vi "SP_OEE_2_test.vi"() -> ()   [LabVIEW 2017] (continued)
                            n1032 = call "Stack_holderwise_total_bd_count_&_duration.vi"("Refnum in"=w5667, "BREAKDOWN_STK_HOLD_ID"=5, "condition"=w5661, "Form Date"=w5664, "To Date"=w5665, "error in (no error)"=w5669) -> ("Refnum out"=w5666:T2, "Count out"=w5663:string[], "appended array"=w5662:dbl[], "error out"=w5668:errorcluster)  [unwired: 6 in]
                          }
                          frame Enabled {
                          }
                        }
                        n1033 = call "NUMERIC TO STRING.vi"("appended array"=w5641) -> ("Array"=w5640:string[])  [unwired: 4 in]
                        n1034 = call "Insert_empty_element_with_zero.vi"("searched date"=w5645, "fixed date"=w5643) -> ("O/P"=w5644:string[])  [unwired: 9 in]
                        n1035 = call "Insert_empty_element_with_zero.vi"("searched date"=w5640, "fixed date"=w5643) -> ("O/P"=w5642:string[])  [unwired: 9 in]
                      }
                      frame #6 {
                        n1036 = call "String to numeric.vi"("Array"=w5683) -> ("Array 2"=w5682:dbl[])  [unwired: 4 in]
                        n1037 = call "String to numeric.vi"("Array"=w5681) -> ("Array 2"=w5680:dbl[])  [unwired: 4 in]
                        n1038 = call "String to numeric.vi"("Array"=w5679) -> ("Array 2"=w5678:dbl[])  [unwired: 4 in]
                        n1039 = call "String to numeric.vi"("Array"=w5677) -> ("Array 2"=w5676:dbl[])  [unwired: 4 in]
                        n1040 = call "String to numeric.vi"("Array"=w5675) -> ("Array 2"=w5674:dbl[])  [unwired: 4 in]
                        n1041 = Decimal String To Number(string=w5688) -> (number=w5707:i32[])  [unwired: 2 in, 1 out]
                        n1042 = Decimal String To Number(string=w5689) -> (number=w5708:i32[])  [unwired: 2 in, 1 out]
                        n1043 = Decimal String To Number(string=w5690) -> (number=w5709:i32[])  [unwired: 2 in, 1 out]
                        n1044 = Decimal String To Number(string=w5691) -> (number=w5710:i32[])  [unwired: 2 in, 1 out]
                        n1045 = Decimal String To Number(string=w5692) -> (number=w5705:i32[])  [unwired: 2 in, 1 out]
                        n1046 = Compound Arithmetic op=ADD(w5682, w5680, w5678, w5676, w5674) -> (w5685:dbl[])
                        n1047 = Build Array(w5683) -> (w5704:string[][])
                        n1048 = Build Array(w5681) -> (w5703:string[][])
                        n1049 = Build Array(w5679) -> (w5702:string[][])
                        n1050 = Build Array(w5677) -> (w5701:string[][])
                        n1051 = Build Array(w5675) -> (w5700:string[][])
                        n1052 = Number To Fractional String(number=w5685, precision (6)=i16 2) -> (F-format string=w5684:string[])  [unwired: 2 in]
                        n1053 = Compound Arithmetic op=ADD(w5707, w5708, w5709, w5710, w5705) -> (w5711:i32[])
                        n1054 = Transpose 2D Array(2D array=w5704) -> (transposed array=w5698:string[][])
                        n1055 = Transpose 2D Array(2D array=w5703) -> (transposed array=w5697:string[][])
                        n1056 = Transpose 2D Array(2D array=w5702) -> (transposed array=w5696:string[][])
                        n1057 = Transpose 2D Array(2D array=w5701) -> (transposed array=w5695:string[][])
                        n1058 = Transpose 2D Array(2D array=w5700) -> (transposed array=w5694:string[][])
                        n1059 = Number To Decimal String(number=w5711) -> (decimal integer string=w5706:string[])  [unwired: 1 in]
                        n1060 = Build Array(w5684) -> (w5687:string[][])
                        n1061 = Transpose 2D Array(2D array=w5687) -> (transposed array=w5693:string[][])
                      }
                      frame #7 {
                        w5715 = string[] [""]
                        n1062 = Insert Into Array(array=w5724, index (col)=1 ("disabled index (col)"), new element #1=w5715, new element #2=w5715, new element #3=w5715, new element #4=w5715, new element #5=w5714, new element #6=w5716, new element #7=w5715, new element #8=w5715, new element #9=w5715, new element #10=w5715, new element #11=w5717, new element #12=w5718) -> (w5720:string[][])  [unwired: 1 in]
                        n1063 = call "flot graph for month n year.vi"("BD Date"=w5721, "error in (no error)"=w5723, "Count total"=w5717) -> ("error out"=w5722:errorcluster, "Run-Time Status"=w5719:cluster{"Array 2":timestamp[], dbl[]})  [unwired: 7 in]
                        n1064 = local write "Run-Time Status"(w5719) -> ()
                        n1065 = local write "Table"(w5720) -> ()
                      }
                    }
                  }
                  frame "3" {
                    n1066 = flat-sequence {
                      tunnel: w5735 -> [w5849]
                      tunnel: w5734 -> [w5847]
                      tunnel: [w5833] -> w5825
                      tunnel: [w5848] -> w5824
                      tunnel: w5733 -> [_]
                      tunnel: [w5852] -> w5823
                      tunnel: [w5832] -> w5822
                      tunnel: [w5831] -> w5821
                      tunnel: [w5830] -> w5820
                      tunnel: w5732 -> [w5832]
                      tunnel: w5731 -> [w5831]
                      tunnel: ["Where BREAKDOWN_DATE between '%s'and '%s' and BREAKDOWN_STK_HOLD_ID ='%d' and  SHIFT_ID = '%d' "] -> w5819
                      tunnel: [w5830] -> w5818
                      tunnel: w5730 -> [w5826]
                      tunnel: [w5826] -> w5729
                      tunnel: w5825 -> [w5913]
                      tunnel: w5824 -> [w5915]
                      tunnel: w5823 -> [w5911]
                      tunnel: w5822 -> [w5910]
                      tunnel: w5821 -> [w5909]
                      tunnel: [w5912] -> w5817
                      tunnel: [w5914] -> w5816
                      tunnel: [w5911] -> w5815
                      tunnel: [w5901] -> w5814
                      tunnel: [w5907] -> w5813
                      tunnel: [w5910] -> w5812
                      tunnel: [w5909] -> w5811
                      tunnel: w5820 -> [w5906]
                      tunnel: [w5906] -> w5810
                      tunnel: w5819 -> [w5903]
                      tunnel: [w5903] -> w5809
                      tunnel: [w5902] -> w5808
                      tunnel: w5818 -> [w5902]
                      tunnel: w5729 -> [w5900]
                      tunnel: [w5899] -> w5728
                      tunnel: w5817 -> [w5945]
                      tunnel: w5816 -> [w5943]
                      tunnel: w5815 -> [w5948]
                      tunnel: w5814 -> [w5947]
                      tunnel: w5813 -> [w5946]
                      tunnel: w5812 -> [w5941]
                      tunnel: w5811 -> [w5940]
                      tunnel: [w5948] -> w5807
                      tunnel: [w5947] -> w5806
                      tunnel: [w5946] -> w5805
                      tunnel: [w5944] -> w5804
                      tunnel: [w5938] -> w5803
                      tunnel: [w5937] -> w5802
                      tunnel: [w5942] -> w5801
                      tunnel: [w5941] -> w5800
                      tunnel: [w5940] -> w5799
                      tunnel: w5810 -> [w5936]
                      tunnel: [w5936] -> w5798
                      tunnel: w5809 -> [w5933]
                      tunnel: [w5933] -> w5797
                      tunnel: [w5932] -> w5796
                      tunnel: w5808 -> [w5932]
                      tunnel: w5728 -> [w5931]
                      tunnel: [w5930] -> w5727
                      tunnel: w5807 -> [w5983]
                      tunnel: w5806 -> [w5982]
                      tunnel: w5805 -> [w5981]
                      tunnel: w5804 -> [w5978]
                      tunnel: w5803 -> [w5980]
                      tunnel: w5802 -> [w5979]
                      tunnel: w5801 -> [w5976]
                      tunnel: w5800 -> [w5974]
                      tunnel: w5799 -> [w5973]
                      tunnel: [w5983] -> w5795
                      tunnel: [w5982] -> w5794
                      tunnel: [w5981] -> w5793
                      tunnel: [w5980] -> w5792
                      tunnel: [w5979] -> w5791
                      tunnel: [w5977] -> w5790
                      tunnel: [w5971] -> w5789
                      tunnel: [w5970] -> w5788
                      tunnel: [w5975] -> w5787
                      tunnel: [w5974] -> w5786
                      tunnel: [w5973] -> w5785
                      tunnel: w5798 -> [w5969]
                      tunnel: [w5969] -> w5784
                      tunnel: w5797 -> [w5966]
                      tunnel: [w5966] -> w5783
                      tunnel: [w5965] -> w5782
                      tunnel: w5796 -> [w5965]
                      tunnel: w5727 -> [w5963]
                      tunnel: w5795 -> [w6004]
                      tunnel: w5794 -> [w6003]
                      tunnel: w5793 -> [w6002]
                      tunnel: w5792 -> [w6001]
                      tunnel: w5791 -> [w6000]
                      tunnel: w5790 -> [w5997]
                      tunnel: w5789 -> [w5999]
                      tunnel: w5788 -> [w5998]
                      tunnel: w5787 -> [w5996]
                      tunnel: w5786 -> [w5993]
                      tunnel: w5785 -> [w5992]
                      tunnel: [w6004] -> w5781
                      tunnel: [w6003] -> w5780
                      tunnel: [w6002] -> w5779
                      tunnel: [w6001] -> w5778
                      tunnel: [w6000] -> w5777
                      tunnel: [w5999] -> w5776
                      tunnel: [w5998] -> w5775
                      tunnel: [w5995] -> w5774
                      tunnel: [w5994] -> w5773
                      tunnel: [w5990] -> w5772
                      tunnel: [w5989] -> w5771
                      tunnel: [w5993] -> w5770
                      tunnel: [w5992] -> w5769
                      tunnel: w5784 -> [w5988]
                      tunnel: [w5988] -> w5768
                      tunnel: w5783 -> [w5985]
                      tunnel: [w5985] -> w5767
                      tunnel: [w5984] -> w5766
                      tunnel: w5782 -> [w5984]
                      tunnel: w5781 -> [w6039]
                      tunnel: w5780 -> [w6038]
                      tunnel: w5779 -> [w6037]
                      tunnel: w5778 -> [w6036]
                      tunnel: w5777 -> [w6035]
                      tunnel: w5776 -> [w6034]
                      tunnel: w5775 -> [w6033]
                      tunnel: w5774 -> [w6028]
                      tunnel: w5773 -> [w6030]
                      tunnel: w5772 -> [w6032]
                      tunnel: w5771 -> [w6031]
                      tunnel: w5770 -> [w6025]
                      tunnel: w5769 -> [w6026]
                      tunnel: [w6039] -> w5765
                      tunnel: [w6038] -> w5764
                      tunnel: [w6037] -> w5763
                      tunnel: [w6036] -> w5762
                      tunnel: [w6035] -> w5761
                      tunnel: [w6034] -> w5760
                      tunnel: [w6033] -> w5759
                      tunnel: [w6032] -> w5758
                      tunnel: [w6031] -> w5757
                      tunnel: [w6029] -> w5756
                      tunnel: [w6027] -> w5755
                      tunnel: [w6023] -> w5754
                      tunnel: [w6021] -> w5753
                      tunnel: w5768 -> [w6022]
                      tunnel: w5767 -> [w6018]
                      tunnel: [w6017] -> w5752
                      tunnel: w5766 -> [w6017]
                      tunnel: w5765 -> [w6078]
                      tunnel: w5764 -> [w6071]
                      tunnel: w5763 -> [w6062]
                      tunnel: w5762 -> [w6070]
                      tunnel: w5761 -> [w6060]
                      tunnel: w5760 -> [w6069]
                      tunnel: w5759 -> [w6058]
                      tunnel: w5758 -> [w6068]
                      tunnel: w5757 -> [w6056]
                      tunnel: w5756 -> [w6092]
                      tunnel: w5755 -> [w6091]
                      tunnel: w5754 -> [w6067]
                      tunnel: w5753 -> [w6054]
                      tunnel: [w6092] -> w5751
                      tunnel: [w6091] -> w5750
                      tunnel: [w6085] -> w5749
                      tunnel: [w6078] -> w5748
                      tunnel: [w6077] -> w5747
                      tunnel: [w6076] -> w5746
                      tunnel: [w6075] -> w5745
                      tunnel: [w6074] -> w5744
                      tunnel: [w6073] -> w5743
                      tunnel: [w6072] -> w5742
                      tunnel: [w6071] -> w5741
                      tunnel: [w6070] -> w5740
                      tunnel: [w6069] -> w5739
                      tunnel: [w6068] -> w5738
                      tunnel: [w6067] -> w5737
                      tunnel: [w6052] -> w5736
                      tunnel: w5752 -> [w6052]
                      tunnel: [w6105] -> _
                      tunnel: [w6101] -> _
                      tunnel: w5751 -> [w6102]
                      tunnel: w5750 -> [w6105]
                      tunnel: w5749 -> [w6096]
                      tunnel: w5748 -> [w6103]
                      tunnel: w5747 -> [_]
                      tunnel: w5746 -> [_]
                      tunnel: w5745 -> [w6095]
                      tunnel: w5744 -> [_]
                      tunnel: w5743 -> [_]
                      tunnel: w5742 -> [w6097]
                      tunnel: w5741 -> [_]
                      tunnel: w5740 -> [_]
                      tunnel: w5739 -> [w6093]
                      tunnel: w5738 -> [_]
                      tunnel: w5737 -> [_]
                      tunnel: w5736 -> [w6100]
                      frame #0 {
                        w5840 = "%Y-%m-%d" ("time format string (%c)")
                        n1067 = Decimal String To Number(string=w5826) -> (number=w5827:i32)  [unwired: 2 in, 1 out]
                        n1068 = property on="Table" class="Tbl (strict)"("Visible"=TRUE) -> ()  [unwired: 2 in, 2 out]
                        n1069 = Format Date/Time String(time format string (%c)=w5840, seconds (now)=w5832) -> (date/time string=w5841:string)  [unwired: 1 in]
                        n1070 = Format Date/Time String(time format string (%c)=w5840, seconds (now)=w5831) -> (date/time string=w5839:string)  [unwired: 1 in]
                        n1071 = Format Into String(format string="Where BREAKDOWN_DATE between '%s' and '%s' and  SHIFT_ID = '%d'  ", w5841, w5839, w5827) -> (resulting string=w5838:string)  [unwired: 2 in, 1 out]
                        n1072 = call <vilib>:"DB Tools Select Data.vi"("condition"=w5838, "error in (no error)"=w5847, "columns"=string[] ["BREAKDOWN_DATE"], "table"="STATION_1_LOG_HISTORY", "connection reference"=w5849) -> ("error out"=w5834:errorcluster, "data"=w5837:variant[][], "connection reference out"=w5848:T2)  [unwired: 1 in]
                        n1073 = property on="Table 2" class="Tbl (strict)"("Visible"=FALSE) -> ()  [unwired: 2 in, 2 out]
                        n1074 = xnode "Database Variant To Data"("database variant"=w5837, "error in (no error)"=w5834, "type"=string[][] [] ("Elements Found")) -> ("data"=w5835:string[][], "error out"=w5833:errorcluster)
                        n1075 = Index Array(array=w5835, index (col)=0 ("disabled index (col)")) -> (element=w5843:string[])  [unwired: 1 in]
                        n1076 = call "Search_1d_array_element.vi"("Count in"=string[] [] ("Elements Found"), "BD Date"=w5843, "Elements Found in"=string[] [] ("Elements Found")) -> ("Elements Found out"=w5830:string[])  [unwired: 4 in, 2 out]
                        n1077 = Build Array(w5830) -> (w5853:string[][])
                        n1078 = Transpose 2D Array(2D array=w5853) -> (transposed array=w5852:string[][])
                      }
                      frame #1 {
                        n1079 = disable-structure shown="Enabled" {
                          disable-tunnel: w5915 -> [w5926 w5928]
                          disable-tunnel: [w5925 w5928] -> w5914
                          disable-tunnel: w5913 -> [w5924 w5929]
                          disable-tunnel: [w5923 w5929] -> w5912
                          disable-tunnel: w5910 -> [w5921 _]
                          disable-tunnel: w5909 -> [w5920 _]
                          disable-tunnel: [w5919 _] -> w5908
                          disable-tunnel: [w5918 _] -> w5905
                          disable-tunnel: w5903 -> [w5917 _]
                          disable-tunnel: w5900 -> [w5916 w5927]
                          disable-tunnel: [_ w5927] -> w5899
                          frame Disabled {
                            n1080 = call "Stack_holderwise_total_bd_count_&_duration_2.vi"("Refnum in"=w5926, "BREAKDOWN_STK_HOLD_ID"=1, "condition"=w5917, "Form Date"=w5921, "To Date"=w5920, "error in (no error)"=w5924, "Shift"=w5916) -> ("Refnum out"=w5925:T2, "Count out"=w5919:string[], "appended array"=w5918:dbl[], "error out"=w5923:errorcluster)  [unwired: 5 in]
                          }
                          frame Enabled {
                          }
                        }
                        n1081 = call "NUMERIC TO STRING.vi"("appended array"=w5905) -> ("Array"=w5904:string[])  [unwired: 4 in]
                        n1082 = call "Insert_empty_element_with_zero.vi"("searched date"=w5908, "fixed date"=w5906) -> ("O/P"=w5901:string[])  [unwired: 9 in]
                        n1083 = call "Insert_empty_element_with_zero.vi"("searched date"=w5904, "fixed date"=w5906) -> ("O/P"=w5907:string[])  [unwired: 9 in]
                      }
                      frame #2 {
                        n1084 = disable-structure shown="Enabled" {
                          disable-tunnel: w5945 -> [w5959 w5961]
                          disable-tunnel: [w5958 w5961] -> w5944
                          disable-tunnel: w5943 -> [w5957 w5962]
                          disable-tunnel: [w5956 w5962] -> w5942
                          disable-tunnel: w5941 -> [w5955 _]
                          disable-tunnel: w5940 -> [w5954 _]
                          disable-tunnel: [w5953 _] -> w5939
                          disable-tunnel: [w5952 _] -> w5935
                          disable-tunnel: w5933 -> [w5951 _]
                          disable-tunnel: w5931 -> [w5949 w5960]
                          disable-tunnel: [_ w5960] -> w5930
                          frame Disabled {
                            n1085 = call "Stack_holderwise_total_bd_count_&_duration_2.vi"("Refnum in"=w5957, "BREAKDOWN_STK_HOLD_ID"=2, "condition"=w5951, "Form Date"=w5955, "To Date"=w5954, "error in (no error)"=w5959, "Shift"=w5949) -> ("Refnum out"=w5956:T2, "Count out"=w5953:string[], "appended array"=w5952:dbl[], "error out"=w5958:errorcluster)  [unwired: 5 in]
                          }
                          frame Enabled {
                          }
                        }
                        n1086 = call "Insert_empty_element_with_zero.vi"("searched date"=w5939, "fixed date"=w5936) -> ("O/P"=w5938:string[])  [unwired: 9 in]
                        n1087 = call "NUMERIC TO STRING.vi"("appended array"=w5935) -> ("Array"=w5934:string[])  [unwired: 4 in]
                        n1088 = call "Insert_empty_element_with_zero.vi"("searched date"=w5934, "fixed date"=w5936) -> ("O/P"=w5937:string[])  [unwired: 9 in]
                      }
                      frame #3 {
                        n1089 = call "Stack_holderwise_total_bd_count_&_duration_2.vi"("Refnum in"=w5976, "BREAKDOWN_STK_HOLD_ID"=3, "condition"=w5966, "Form Date"=w5974, "To Date"=w5973, "error in (no error)"=w5978, "Shift"=w5963) -> ("Refnum out"=w5975:T2, "Count out"=w5972:string[], "appended array"=w5968:dbl[], "error out"=w5977:errorcluster)  [unwired: 5 in]
                        n1090 = call "Insert_empty_element_with_zero.vi"("searched date"=w5972, "fixed date"=w5969) -> ("O/P"=w5971:string[])  [unwired: 9 in]
                        n1091 = call "NUMERIC TO STRING.vi"("appended array"=w5968) -> ("Array"=w5967:string[])  [unwired: 4 in]
                        n1092 = call "Insert_empty_element_with_zero.vi"("searched date"=w5967, "fixed date"=w5969) -> ("O/P"=w5970:string[])  [unwired: 9 in]
                      }
                      frame #4 {
                        n1093 = disable-structure shown="Enabled" {
                          disable-tunnel: w5997 -> [w6013 w6016]
                          disable-tunnel: w5996 -> [w6012 w6015]
                          disable-tunnel: [w6011 w6015] -> w5995
                          disable-tunnel: [w6010 w6016] -> w5994
                          disable-tunnel: w5993 -> [w6009 _]
                          disable-tunnel: w5992 -> [w6008 _]
                          disable-tunnel: [w6007 _] -> w5991
                          disable-tunnel: [w6006 _] -> w5987
                          disable-tunnel: w5985 -> [w6005 _]
                          frame Disabled {
                            n1094 = call "Stack_holderwise_total_bd_count_&_duration.vi"("Refnum in"=w6012, "BREAKDOWN_STK_HOLD_ID"=4, "condition"=w6005, "Form Date"=w6009, "To Date"=w6008, "error in (no error)"=w6013) -> ("Refnum out"=w6011:T2, "Count out"=w6007:string[], "appended array"=w6006:dbl[], "error out"=w6010:errorcluster)  [unwired: 6 in]
                          }
                          frame Enabled {
                          }
                        }
                        n1095 = call "Insert_empty_element_with_zero.vi"("searched date"=w5991, "fixed date"=w5988) -> ("O/P"=w5990:string[])  [unwired: 9 in]
                        n1096 = call "NUMERIC TO STRING.vi"("appended array"=w5987) -> ("Array"=w5986:string[])  [unwired: 4 in]
                        n1097 = call "Insert_empty_element_with_zero.vi"("searched date"=w5986, "fixed date"=w5988) -> ("O/P"=w5989:string[])  [unwired: 9 in]
                      }
                      frame #5 {
                        n1098 = disable-structure shown="Enabled" {
                          disable-tunnel: w6030 -> [w6048 w6051]
                          disable-tunnel: [w6047 w6051] -> w6029
                          disable-tunnel: w6028 -> [w6046 w6050]
                          disable-tunnel: [w6045 w6050] -> w6027
                          disable-tunnel: w6026 -> [w6044 _]
                          disable-tunnel: w6025 -> [w6043 _]
                          disable-tunnel: [w6042 _] -> w6024
                          disable-tunnel: [w6041 _] -> w6020
                          disable-tunnel: w6018 -> [w6040 _]
                          frame Disabled {
                            n1099 = call "Stack_holderwise_total_bd_count_&_duration.vi"("Refnum in"=w6046, "BREAKDOWN_STK_HOLD_ID"=5, "condition"=w6040, "Form Date"=w6043, "To Date"=w6044, "error in (no error)"=w6048) -> ("Refnum out"=w6045:T2, "Count out"=w6042:string[], "appended array"=w6041:dbl[], "error out"=w6047:errorcluster)  [unwired: 6 in]
                          }
                          frame Enabled {
                          }
                        }
                        n1100 = call "NUMERIC TO STRING.vi"("appended array"=w6020) -> ("Array"=w6019:string[])  [unwired: 4 in]
                        n1101 = call "Insert_empty_element_with_zero.vi"("searched date"=w6024, "fixed date"=w6022) -> ("O/P"=w6023:string[])  [unwired: 9 in]
                        n1102 = call "Insert_empty_element_with_zero.vi"("searched date"=w6019, "fixed date"=w6022) -> ("O/P"=w6021:string[])  [unwired: 9 in]
                      }
                      frame #6 {
                        n1103 = call "String to numeric.vi"("Array"=w6062) -> ("Array 2"=w6061:dbl[])  [unwired: 4 in]
                        n1104 = call "String to numeric.vi"("Array"=w6060) -> ("Array 2"=w6059:dbl[])  [unwired: 4 in]
                        n1105 = call "String to numeric.vi"("Array"=w6058) -> ("Array 2"=w6057:dbl[])  [unwired: 4 in]
                        n1106 = call "String to numeric.vi"("Array"=w6056) -> ("Array 2"=w6055:dbl[])  [unwired: 4 in]
                        n1107 = call "String to numeric.vi"("Array"=w6054) -> ("Array 2"=w6053:dbl[])  [unwired: 4 in]
                        n1108 = Decimal String To Number(string=w6067) -> (number=w6086:i32[])  [unwired: 2 in, 1 out]
                        n1109 = Decimal String To Number(string=w6068) -> (number=w6087:i32[])  [unwired: 2 in, 1 out]
                        n1110 = Decimal String To Number(string=w6069) -> (number=w6088:i32[])  [unwired: 2 in, 1 out]
                        n1111 = Decimal String To Number(string=w6070) -> (number=w6089:i32[])  [unwired: 2 in, 1 out]
                        n1112 = Decimal String To Number(string=w6071) -> (number=w6084:i32[])  [unwired: 2 in, 1 out]
                        n1113 = Compound Arithmetic op=ADD(w6061, w6059, w6057, w6055, w6053) -> (w6064:dbl[])
                        n1114 = Build Array(w6062) -> (w6083:string[][])
                        n1115 = Build Array(w6060) -> (w6082:string[][])
                        n1116 = Build Array(w6058) -> (w6081:string[][])
                        n1117 = Build Array(w6056) -> (w6080:string[][])
                        n1118 = Build Array(w6054) -> (w6079:string[][])
                        n1119 = Number To Fractional String(number=w6064, precision (6)=i16 2) -> (F-format string=w6063:string[])  [unwired: 2 in]
                        n1120 = Compound Arithmetic op=ADD(w6086, w6087, w6088, w6089, w6084) -> (w6090:i32[])
                        n1121 = Transpose 2D Array(2D array=w6083) -> (transposed array=w6077:string[][])
                        n1122 = Transpose 2D Array(2D array=w6082) -> (transposed array=w6076:string[][])
                        n1123 = Transpose 2D Array(2D array=w6081) -> (transposed array=w6075:string[][])
                        n1124 = Transpose 2D Array(2D array=w6080) -> (transposed array=w6074:string[][])
                        n1125 = Transpose 2D Array(2D array=w6079) -> (transposed array=w6073:string[][])
                        n1126 = Number To Decimal String(number=w6090) -> (decimal integer string=w6085:string[])  [unwired: 1 in]
                        n1127 = Build Array(w6063) -> (w6066:string[][])
                        n1128 = Transpose 2D Array(2D array=w6066) -> (transposed array=w6072:string[][])
                      }
                      frame #7 {
                        w6094 = string[] [""]
                        n1129 = Insert Into Array(array=w6103, index (col)=1 ("disabled index (col)"), new element #1=w6094, new element #2=w6094, new element #3=w6094, new element #4=w6094, new element #5=w6093, new element #6=w6095, new element #7=w6094, new element #8=w6094, new element #9=w6094, new element #10=w6094, new element #11=w6096, new element #12=w6097) -> (w6099:string[][])  [unwired: 1 in]
                        n1130 = call "flot graph for month n year.vi"("BD Date"=w6100, "error in (no error)"=w6102, "Count total"=w6096) -> ("error out"=w6101:errorcluster, "Run-Time Status"=w6098:cluster{"Array 2":timestamp[], dbl[]})  [unwired: 7 in]
                        n1131 = local write "Run-Time Status"(w6098) -> ()
                        n1132 = local write "Table"(w6099) -> ()
                      }
                    }
                  }
                  frame "all" {
                  }
                }
              }
              frame "Quality" {
                n1133 = local read "Shift"() -> (w6106:string)
                n1134 = case shown="\"3\"" w6106 {
                  selector: w6106 -> [_ w6480 w6864 w7248 _]
                  tunnel: w6111 -> [w6116 w6485 w6869 w7253 _]
                  tunnel: w6110 -> [w6115 w6484 w6868 w7252 _]
                  tunnel: w6109 -> [w6114 w6483 w6867 w7251 _]
                  tunnel: w6108 -> [w6113 w6482 w6866 w7250 _]
                  tunnel: w6107 -> [w6112 w6481 w6865 w7249 _]
                  frame "ALL", Default {
                    n1135 = flat-sequence {
                      tunnel: w6116 -> [w6228]
                      tunnel: w6115 -> [w6226]
                      tunnel: [w6212] -> w6206
                      tunnel: [w6227] -> w6205
                      tunnel: w6114 -> [_]
                      tunnel: [w6231] -> w6204
                      tunnel: [w6211] -> w6203
                      tunnel: [w6210] -> w6202
                      tunnel: [w6208] -> w6201
                      tunnel: w6113 -> [w6211]
                      tunnel: w6112 -> [w6210]
                      tunnel: ["Where BREAKDOWN_DATE between '%s'and '%s' and BREAKDOWN_STK_HOLD_ID ='%d'  "] -> w6200
                      tunnel: [w6208] -> w6199
                      tunnel: w6206 -> [w6290]
                      tunnel: w6205 -> [w6292]
                      tunnel: w6204 -> [w6288]
                      tunnel: w6203 -> [w6287]
                      tunnel: w6202 -> [w6286]
                      tunnel: [w6289] -> w6198
                      tunnel: [w6291] -> w6197
                      tunnel: [w6288] -> w6196
                      tunnel: [w6278] -> w6195
                      tunnel: [w6284] -> w6194
                      tunnel: [w6287] -> w6193
                      tunnel: [w6286] -> w6192
                      tunnel: w6201 -> [w6283]
                      tunnel: [w6283] -> w6191
                      tunnel: w6200 -> [w6280]
                      tunnel: [w6280] -> w6190
                      tunnel: [w6279] -> w6189
                      tunnel: w6199 -> [w6279]
                      tunnel: w6198 -> [w6318]
                      tunnel: w6197 -> [w6316]
                      tunnel: w6196 -> [w6321]
                      tunnel: w6195 -> [w6320]
                      tunnel: w6194 -> [w6319]
                      tunnel: w6193 -> [w6314]
                      tunnel: w6192 -> [w6313]
                      tunnel: [w6321] -> w6188
                      tunnel: [w6320] -> w6187
                      tunnel: [w6319] -> w6186
                      tunnel: [w6317] -> w6185
                      tunnel: [w6311] -> w6184
                      tunnel: [w6310] -> w6183
                      tunnel: [w6315] -> w6182
                      tunnel: [w6314] -> w6181
                      tunnel: [w6313] -> w6180
                      tunnel: w6191 -> [w6309]
                      tunnel: [w6309] -> w6179
                      tunnel: w6190 -> [w6306]
                      tunnel: [w6306] -> w6178
                      tunnel: [w6305] -> w6177
                      tunnel: w6189 -> [w6305]
                      tunnel: w6188 -> [w6352]
                      tunnel: w6187 -> [w6351]
                      tunnel: w6186 -> [w6350]
                      tunnel: w6185 -> [w6347]
                      tunnel: w6184 -> [w6349]
                      tunnel: w6183 -> [w6348]
                      tunnel: w6182 -> [w6345]
                      tunnel: w6181 -> [w6343]
                      tunnel: w6180 -> [w6342]
                      tunnel: [w6352] -> w6176
                      tunnel: [w6351] -> w6175
                      tunnel: [w6350] -> w6174
                      tunnel: [w6349] -> w6173
                      tunnel: [w6348] -> w6172
                      tunnel: [w6346] -> w6171
                      tunnel: [w6340] -> w6170
                      tunnel: [w6339] -> w6169
                      tunnel: [w6344] -> w6168
                      tunnel: [w6343] -> w6167
                      tunnel: [w6342] -> w6166
                      tunnel: w6179 -> [w6338]
                      tunnel: [w6338] -> w6165
                      tunnel: w6178 -> [w6335]
                      tunnel: [w6335] -> w6164
                      tunnel: [w6334] -> w6163
                      tunnel: w6177 -> [w6334]
                      tunnel: w6176 -> [w6386]
                      tunnel: w6175 -> [w6385]
                      tunnel: w6174 -> [w6384]
                      tunnel: w6173 -> [w6383]
                      tunnel: w6172 -> [w6382]
                      tunnel: w6171 -> [w6379]
                      tunnel: w6170 -> [w6381]
                      tunnel: w6169 -> [w6380]
                      tunnel: w6168 -> [w6378]
                      tunnel: w6167 -> [w6375]
                      tunnel: w6166 -> [w6374]
                      tunnel: [w6386] -> w6162
                      tunnel: [w6385] -> w6161
                      tunnel: [w6384] -> w6160
                      tunnel: [w6383] -> w6159
                      tunnel: [w6382] -> w6158
                      tunnel: [w6381] -> w6157
                      tunnel: [w6380] -> w6156
                      tunnel: [w6377] -> w6155
                      tunnel: [w6376] -> w6154
                      tunnel: [w6372] -> w6153
                      tunnel: [w6371] -> w6152
                      tunnel: [w6375] -> w6151
                      tunnel: [w6374] -> w6150
                      tunnel: w6165 -> [w6370]
                      tunnel: [w6370] -> w6149
                      tunnel: w6164 -> [w6367]
                      tunnel: [w6367] -> w6148
                      tunnel: [w6366] -> w6147
                      tunnel: w6163 -> [w6366]
                      tunnel: w6162 -> [w6409]
                      tunnel: w6161 -> [w6408]
                      tunnel: w6160 -> [w6407]
                      tunnel: w6159 -> [w6406]
                      tunnel: w6158 -> [w6405]
                      tunnel: w6157 -> [w6404]
                      tunnel: w6156 -> [w6403]
                      tunnel: w6155 -> [w6398]
                      tunnel: w6154 -> [w6400]
                      tunnel: w6153 -> [w6402]
                      tunnel: w6152 -> [w6401]
                      tunnel: w6151 -> [w6395]
                      tunnel: w6150 -> [w6396]
                      tunnel: [w6409] -> w6146
                      tunnel: [w6408] -> w6145
                      tunnel: [w6407] -> w6144
                      tunnel: [w6406] -> w6143
                      tunnel: [w6405] -> w6142
                      tunnel: [w6404] -> w6141
                      tunnel: [w6403] -> w6140
                      tunnel: [w6402] -> w6139
                      tunnel: [w6401] -> w6138
                      tunnel: [w6399] -> w6137
                      tunnel: [w6397] -> w6136
                      tunnel: [w6393] -> w6135
                      tunnel: [w6391] -> w6134
                      tunnel: w6149 -> [w6392]
                      tunnel: w6148 -> [w6388]
                      tunnel: [w6387] -> w6133
                      tunnel: w6147 -> [w6387]
                      tunnel: w6146 -> [w6448]
                      tunnel: w6145 -> [w6441]
                      tunnel: w6144 -> [w6432]
                      tunnel: w6143 -> [w6440]
                      tunnel: w6142 -> [w6430]
                      tunnel: w6141 -> [w6439]
                      tunnel: w6140 -> [w6428]
                      tunnel: w6139 -> [w6438]
                      tunnel: w6138 -> [w6426]
                      tunnel: w6137 -> [w6462]
                      tunnel: w6136 -> [w6461]
                      tunnel: w6135 -> [w6437]
                      tunnel: w6134 -> [w6424]
                      tunnel: [w6462] -> w6132
                      tunnel: [w6461] -> w6131
                      tunnel: [w6455] -> w6130
                      tunnel: [w6448] -> w6129
                      tunnel: [w6447] -> w6128
                      tunnel: [w6446] -> w6127
                      tunnel: [w6445] -> w6126
                      tunnel: [w6444] -> w6125
                      tunnel: [w6443] -> w6124
                      tunnel: [w6442] -> w6123
                      tunnel: [w6441] -> w6122
                      tunnel: [w6440] -> w6121
                      tunnel: [w6439] -> w6120
                      tunnel: [w6438] -> w6119
                      tunnel: [w6437] -> w6118
                      tunnel: [w6422] -> w6117
                      tunnel: w6133 -> [w6422]
                      tunnel: [w6475] -> _
                      tunnel: [w6471] -> _
                      tunnel: w6132 -> [w6472]
                      tunnel: w6131 -> [w6475]
                      tunnel: w6130 -> [w6466]
                      tunnel: w6129 -> [w6473]
                      tunnel: w6128 -> [_]
                      tunnel: w6127 -> [_]
                      tunnel: w6126 -> [_]
                      tunnel: w6125 -> [w6463]
                      tunnel: w6124 -> [_]
                      tunnel: w6123 -> [w6467]
                      tunnel: w6122 -> [_]
                      tunnel: w6121 -> [_]
                      tunnel: w6120 -> [_]
                      tunnel: w6119 -> [w6464]
                      tunnel: w6118 -> [_]
                      tunnel: w6117 -> [w6470]
                      frame #0 {
                        w6219 = "%Y-%m-%d" ("time format string (%c)")
                        n1136 = property on="Table" class="Tbl (strict)"("Visible"=TRUE) -> ()  [unwired: 2 in, 2 out]
                        n1137 = Format Date/Time String(time format string (%c)=w6219, seconds (now)=w6211) -> (date/time string=w6220:string)  [unwired: 1 in]
                        n1138 = Format Date/Time String(time format string (%c)=w6219, seconds (now)=w6210) -> (date/time string=w6218:string)  [unwired: 1 in]
                        n1139 = Format Into String(format string="Where BREAKDOWN_DATE between '%s' and '%s' ", w6220, w6218) -> (resulting string=w6217:string)  [unwired: 2 in, 1 out]
                        n1140 = call <vilib>:"DB Tools Select Data.vi"("condition"=w6217, "error in (no error)"=w6226, "columns"=string[] ["BREAKDOWN_DATE"], "table"="STATION_1_LOG_HISTORY", "connection reference"=w6228) -> ("error out"=w6213:errorcluster, "data"=w6216:variant[][], "connection reference out"=w6227:T2)  [unwired: 1 in]
                        n1141 = property on="Table 2" class="Tbl (strict)"("Visible"=FALSE) -> ()  [unwired: 2 in, 2 out]
                        n1142 = xnode "Database Variant To Data"("database variant"=w6216, "error in (no error)"=w6213, "type"=string[][] [] ("Elements Found")) -> ("data"=w6214:string[][], "error out"=w6212:errorcluster)
                        n1143 = Index Array(array=w6214, index (col)=0 ("disabled index (col)")) -> (element=w6222:string[])  [unwired: 1 in]
                        n1144 = call "Search_1d_array_element.vi"("Count in"=string[] [] ("Elements Found"), "BD Date"=w6222, "Elements Found in"=string[] [] ("Elements Found")) -> ("Elements Found out"=w6208:string[])  [unwired: 4 in, 2 out]
                        n1145 = Build Array(w6208) -> (w6232:string[][])
                        n1146 = Transpose 2D Array(2D array=w6232) -> (transposed array=w6231:string[][])
                      }
                      frame #1 {
                        n1147 = disable-structure shown="Enabled" {
                          disable-tunnel: w6292 -> [w6302 w6303]
                          disable-tunnel: [w6301 w6303] -> w6291
                          disable-tunnel: w6290 -> [w6300 w6304]
                          disable-tunnel: [w6299 w6304] -> w6289
                          disable-tunnel: w6287 -> [w6297 _]
                          disable-tunnel: w6286 -> [w6296 _]
                          disable-tunnel: [w6295 _] -> w6285
                          disable-tunnel: [w6294 _] -> w6282
                          disable-tunnel: w6280 -> [w6293 _]
                          frame Disabled {
                            n1148 = call "Stack_holderwise_total_bd_count_&_duration.vi"("Refnum in"=w6302, "BREAKDOWN_STK_HOLD_ID"=1, "condition"=w6293, "Form Date"=w6297, "To Date"=w6296, "error in (no error)"=w6300) -> ("Refnum out"=w6301:T2, "Count out"=w6295:string[], "appended array"=w6294:dbl[], "error out"=w6299:errorcluster)  [unwired: 6 in]
                          }
                          frame Enabled {
                          }
                        }
                        n1149 = call "NUMERIC TO STRING.vi"("appended array"=w6282) -> ("Array"=w6281:string[])  [unwired: 4 in]
                        n1150 = call "Insert_empty_element_with_zero.vi"("searched date"=w6285, "fixed date"=w6283) -> ("O/P"=w6278:string[])  [unwired: 9 in]
                        n1151 = call "Insert_empty_element_with_zero.vi"("searched date"=w6281, "fixed date"=w6283) -> ("O/P"=w6284:string[])  [unwired: 9 in]
                      }
                      frame #2 {
                        n1152 = disable-structure shown="Enabled" {
                          disable-tunnel: w6318 -> [w6331 w6333]
                          disable-tunnel: [w6330 w6333] -> w6317
                          disable-tunnel: w6316 -> [w6329 w6332]
                          disable-tunnel: [w6328 w6332] -> w6315
                          disable-tunnel: w6314 -> [w6327 _]
                          disable-tunnel: w6313 -> [w6326 _]
                          disable-tunnel: [w6325 _] -> w6312
                          disable-tunnel: [w6324 _] -> w6308
                          disable-tunnel: w6306 -> [w6323 _]
                          frame Disabled {
                            n1153 = call "Stack_holderwise_total_bd_count_&_duration.vi"("Refnum in"=w6329, "BREAKDOWN_STK_HOLD_ID"=2, "condition"=w6323, "Form Date"=w6327, "To Date"=w6326, "error in (no error)"=w6331) -> ("Refnum out"=w6328:T2, "Count out"=w6325:string[], "appended array"=w6324:dbl[], "error out"=w6330:errorcluster)  [unwired: 6 in]
                          }
                          frame Enabled {
                          }
                        }
                        n1154 = call "Insert_empty_element_with_zero.vi"("searched date"=w6312, "fixed date"=w6309) -> ("O/P"=w6311:string[])  [unwired: 9 in]
                        n1155 = call "NUMERIC TO STRING.vi"("appended array"=w6308) -> ("Array"=w6307:string[])  [unwired: 4 in]
                        n1156 = call "Insert_empty_element_with_zero.vi"("searched date"=w6307, "fixed date"=w6309) -> ("O/P"=w6310:string[])  [unwired: 9 in]
                      }
                      frame #3 {
                        n1157 = disable-structure shown="Enabled" {
                          disable-tunnel: w6347 -> [w6362 w6364]
                          disable-tunnel: [w6361 w6364] -> w6346
                          disable-tunnel: w6345 -> [w6360 w6363]
                          disable-tunnel: [w6359 w6363] -> w6344
                          disable-tunnel: w6343 -> [w6358 _]
                          disable-tunnel: w6342 -> [w6357 _]
                          disable-tunnel: [w6356 _] -> w6341
                          disable-tunnel: [w6355 _] -> w6337
                          disable-tunnel: w6335 -> [w6354 _]
                          frame Disabled {
                            n1158 = call "Stack_holderwise_total_bd_count_&_duration.vi"("Refnum in"=w6360, "BREAKDOWN_STK_HOLD_ID"=3, "condition"=w6354, "Form Date"=w6358, "To Date"=w6357, "error in (no error)"=w6362) -> ("Refnum out"=w6359:T2, "Count out"=w6356:string[], "appended array"=w6355:dbl[], "error out"=w6361:errorcluster)  [unwired: 6 in]
                          }
                          frame Enabled {
                          }
                        }
                        n1159 = call "Insert_empty_element_with_zero.vi"("searched date"=w6341, "fixed date"=w6338) -> ("O/P"=w6340:string[])  [unwired: 9 in]
                        n1160 = call "NUMERIC TO STRING.vi"("appended array"=w6337) -> ("Array"=w6336:string[])  [unwired: 4 in]
                        n1161 = call "Insert_empty_element_with_zero.vi"("searched date"=w6336, "fixed date"=w6338) -> ("O/P"=w6339:string[])  [unwired: 9 in]
                      }
                      frame #4 {
                        n1162 = call "Stack_holderwise_total_bd_count_&_duration.vi"("Refnum in"=w6378, "BREAKDOWN_STK_HOLD_ID"=4, "condition"=w6367, "Form Date"=w6375, "To Date"=w6374, "error in (no error)"=w6379) -> ("Refnum out"=w6377:T2, "Count out"=w6373:string[], "appended array"=w6369:dbl[], "error out"=w6376:errorcluster)  [unwired: 6 in]
                        n1163 = call "Insert_empty_element_with_zero.vi"("searched date"=w6373, "fixed date"=w6370) -> ("O/P"=w6372:string[])  [unwired: 9 in]
                        n1164 = call "NUMERIC TO STRING.vi"("appended array"=w6369) -> ("Array"=w6368:string[])  [unwired: 4 in]
                        n1165 = call "Insert_empty_element_with_zero.vi"("searched date"=w6368, "fixed date"=w6370) -> ("O/P"=w6371:string[])  [unwired: 9 in]
                      }
                      frame #5 {
                        n1166 = disable-structure shown="Enabled" {
                          disable-tunnel: w6400 -> [w6418 w6421]
                          disable-tunnel: [w6417 w6421] -> w6399
                          disable-tunnel: w6398 -> [w6416 w6420]
                          disable-tunnel: [w6415 w6420] -> w6397
                          disable-tunnel: w6396 -> [w6414 _]
                          disable-tunnel: w6395 -> [w6413 _]
                          disable-tunnel: [w6412 _] -> w6394
                          disable-tunnel: [w6411 _] -> w6390
                          disable-tunnel: w6388 -> [w6410 _]
                          frame Disabled {
                            n1167 = call "Stack_holderwise_total_bd_count_&_duration.vi"("Refnum in"=w6416, "BREAKDOWN_STK_HOLD_ID"=5, "condition"=w6410, "Form Date"=w6413, "To Date"=w6414, "error in (no error)"=w6418) -> ("Refnum out"=w6415:T2, "Count out"=w6412:string[], "appended array"=w6411:dbl[], "error out"=w6417:errorcluster)  [unwired: 6 in]
                          }
                          frame Enabled {
                          }
                        }
                        n1168 = call "NUMERIC TO STRING.vi"("appended array"=w6390) -> ("Array"=w6389:string[])  [unwired: 4 in]
                        n1169 = call "Insert_empty_element_with_zero.vi"("searched date"=w6394, "fixed date"=w6392) -> ("O/P"=w6393:string[])  [unwired: 9 in]
                        n1170 = call "Insert_empty_element_with_zero.vi"("searched date"=w6389, "fixed date"=w6392) -> ("O/P"=w6391:string[])  [unwired: 9 in]
                      }
                      frame #6 {
                        n1171 = call "String to numeric.vi"("Array"=w6432) -> ("Array 2"=w6431:dbl[])  [unwired: 4 in]
                        n1172 = call "String to numeric.vi"("Array"=w6430) -> ("Array 2"=w6429:dbl[])  [unwired: 4 in]
                        n1173 = call "String to numeric.vi"("Array"=w6428) -> ("Array 2"=w6427:dbl[])  [unwired: 4 in]
                        n1174 = call "String to numeric.vi"("Array"=w6426) -> ("Array 2"=w6425:dbl[])  [unwired: 4 in]
                        n1175 = call "String to numeric.vi"("Array"=w6424) -> ("Array 2"=w6423:dbl[])  [unwired: 4 in]
                        n1176 = Decimal String To Number(string=w6437) -> (number=w6456:i32[])  [unwired: 2 in, 1 out]
                        n1177 = Decimal String To Number(string=w6438) -> (number=w6457:i32[])  [unwired: 2 in, 1 out]
                        n1178 = Decimal String To Number(string=w6439) -> (number=w6458:i32[])  [unwired: 2 in, 1 out]
                        n1179 = Decimal String To Number(string=w6440) -> (number=w6459:i32[])  [unwired: 2 in, 1 out]
                        n1180 = Decimal String To Number(string=w6441) -> (number=w6454:i32[])  [unwired: 2 in, 1 out]
                        n1181 = Compound Arithmetic op=ADD(w6431, w6429, w6427, w6425, w6423) -> (w6434:dbl[])
                        n1182 = Build Array(w6432) -> (w6453:string[][])
                        n1183 = Build Array(w6430) -> (w6452:string[][])
                        n1184 = Build Array(w6428) -> (w6451:string[][])
                        n1185 = Build Array(w6426) -> (w6450:string[][])
                        n1186 = Build Array(w6424) -> (w6449:string[][])
                        n1187 = Number To Fractional String(number=w6434, precision (6)=i16 2) -> (F-format string=w6433:string[])  [unwired: 2 in]
                        n1188 = Compound Arithmetic op=ADD(w6456, w6457, w6458, w6459, w6454) -> (w6460:i32[])
                        n1189 = Transpose 2D Array(2D array=w6453) -> (transposed array=w6447:string[][])
                        n1190 = Transpose 2D Array(2D array=w6452) -> (transposed array=w6446:string[][])
                        n1191 = Transpose 2D Array(2D array=w6451) -> (transposed array=w6445:string[][])
                        n1192 = Transpose 2D Array(2D array=w6450) -> (transposed array=w6444:string[][])
                        n1193 = Transpose 2D Array(2D array=w6449) -> (transposed array=w6443:string[][])
                        n1194 = Number To Decimal String(number=w6460) -> (decimal integer string=w6455:string[])  [unwired: 1 in]
                        n1195 = Build Array(w6433) -> (w6436:string[][])
                        n1196 = Transpose 2D Array(2D array=w6436) -> (transposed array=w6442:string[][])
                      }
                      frame #7 {
                        w6465 = string[] [""]
                        n1197 = Insert Into Array(array=w6473, index (col)=1 ("disabled index (col)"), new element #1=w6465, new element #2=w6465, new element #3=w6465, new element #4=w6465, new element #5=w6465, new element #6=w6465, new element #7=w6464, new element #8=w6463, new element #9=w6465, new element #10=w6465, new element #11=w6466, new element #12=w6467) -> (w6469:string[][])  [unwired: 1 in]
                        n1198 = call "flot graph for month n year.vi"("BD Date"=w6470, "error in (no error)"=w6472, "Count total"=w6466) -> ("error out"=w6471:errorcluster, "Run-Time Status"=w6468:cluster{"Array 2":timestamp[], dbl[]})  [unwired: 7 in]
                        n1199 = local write "Run-Time Status"(w6468) -> ()
                        n1200 = local write "Table"(w6469) -> ()
                      }
                    }
                  }
                  frame "1" {
                    n1201 = flat-sequence {
                      tunnel: w6485 -> [w6599]
                      tunnel: w6484 -> [w6597]
                      tunnel: [w6583] -> w6575
                      tunnel: [w6598] -> w6574
                      tunnel: w6483 -> [_]
                      tunnel: [w6602] -> w6573
                      tunnel: [w6582] -> w6572
                      tunnel: [w6581] -> w6571
                      tunnel: [w6580] -> w6570
                      tunnel: w6482 -> [w6582]
                      tunnel: w6481 -> [w6581]
                      tunnel: ["Where BREAKDOWN_DATE between '%s'and '%s' and BREAKDOWN_STK_HOLD_ID ='%d' and  SHIFT_ID = '%d' "] -> w6569
                      tunnel: [w6580] -> w6568
                      tunnel: w6480 -> [w6576]
                      tunnel: [w6576] -> w6479
                      tunnel: w6575 -> [w6663]
                      tunnel: w6574 -> [w6665]
                      tunnel: w6573 -> [w6661]
                      tunnel: w6572 -> [w6660]
                      tunnel: w6571 -> [w6659]
                      tunnel: [w6662] -> w6567
                      tunnel: [w6664] -> w6566
                      tunnel: [w6661] -> w6565
                      tunnel: [w6651] -> w6564
                      tunnel: [w6657] -> w6563
                      tunnel: [w6660] -> w6562
                      tunnel: [w6659] -> w6561
                      tunnel: w6570 -> [w6656]
                      tunnel: [w6656] -> w6560
                      tunnel: w6569 -> [w6653]
                      tunnel: [w6653] -> w6559
                      tunnel: [w6652] -> w6558
                      tunnel: w6568 -> [w6652]
                      tunnel: w6479 -> [w6650]
                      tunnel: [w6649] -> w6478
                      tunnel: w6567 -> [w6695]
                      tunnel: w6566 -> [w6693]
                      tunnel: w6565 -> [w6698]
                      tunnel: w6564 -> [w6697]
                      tunnel: w6563 -> [w6696]
                      tunnel: w6562 -> [w6691]
                      tunnel: w6561 -> [w6690]
                      tunnel: [w6698] -> w6557
                      tunnel: [w6697] -> w6556
                      tunnel: [w6696] -> w6555
                      tunnel: [w6694] -> w6554
                      tunnel: [w6688] -> w6553
                      tunnel: [w6687] -> w6552
                      tunnel: [w6692] -> w6551
                      tunnel: [w6691] -> w6550
                      tunnel: [w6690] -> w6549
                      tunnel: w6560 -> [w6686]
                      tunnel: [w6686] -> w6548
                      tunnel: w6559 -> [w6683]
                      tunnel: [w6683] -> w6547
                      tunnel: [w6682] -> w6546
                      tunnel: w6558 -> [w6682]
                      tunnel: w6478 -> [w6681]
                      tunnel: [w6680] -> w6477
                      tunnel: w6557 -> [w6733]
                      tunnel: w6556 -> [w6732]
                      tunnel: w6555 -> [w6731]
                      tunnel: w6554 -> [w6728]
                      tunnel: w6553 -> [w6730]
                      tunnel: w6552 -> [w6729]
                      tunnel: w6551 -> [w6726]
                      tunnel: w6550 -> [w6724]
                      tunnel: w6549 -> [w6723]
                      tunnel: [w6733] -> w6545
                      tunnel: [w6732] -> w6544
                      tunnel: [w6731] -> w6543
                      tunnel: [w6730] -> w6542
                      tunnel: [w6729] -> w6541
                      tunnel: [w6727] -> w6540
                      tunnel: [w6721] -> w6539
                      tunnel: [w6720] -> w6538
                      tunnel: [w6725] -> w6537
                      tunnel: [w6724] -> w6536
                      tunnel: [w6723] -> w6535
                      tunnel: w6548 -> [w6719]
                      tunnel: [w6719] -> w6534
                      tunnel: w6547 -> [w6716]
                      tunnel: [w6716] -> w6533
                      tunnel: [w6715] -> w6532
                      tunnel: w6546 -> [w6715]
                      tunnel: w6477 -> [w6714]
                      tunnel: [w6713] -> w6476
                      tunnel: w6545 -> [w6770]
                      tunnel: w6544 -> [w6769]
                      tunnel: w6543 -> [w6768]
                      tunnel: w6542 -> [w6767]
                      tunnel: w6541 -> [w6766]
                      tunnel: w6540 -> [w6763]
                      tunnel: w6539 -> [w6765]
                      tunnel: w6538 -> [w6764]
                      tunnel: w6537 -> [w6762]
                      tunnel: w6536 -> [w6759]
                      tunnel: w6535 -> [w6758]
                      tunnel: [w6770] -> w6531
                      tunnel: [w6769] -> w6530
                      tunnel: [w6768] -> w6529
                      tunnel: [w6767] -> w6528
                      tunnel: [w6766] -> w6527
                      tunnel: [w6765] -> w6526
                      tunnel: [w6764] -> w6525
                      tunnel: [w6761] -> w6524
                      tunnel: [w6760] -> w6523
                      tunnel: [w6756] -> w6522
                      tunnel: [w6755] -> w6521
                      tunnel: [w6759] -> w6520
                      tunnel: [w6758] -> w6519
                      tunnel: w6534 -> [w6754]
                      tunnel: [w6754] -> w6518
                      tunnel: w6533 -> [w6751]
                      tunnel: [w6751] -> w6517
                      tunnel: [w6750] -> w6516
                      tunnel: w6532 -> [w6750]
                      tunnel: w6476 -> [w6748]
                      tunnel: w6531 -> [w6793]
                      tunnel: w6530 -> [w6792]
                      tunnel: w6529 -> [w6791]
                      tunnel: w6528 -> [w6790]
                      tunnel: w6527 -> [w6789]
                      tunnel: w6526 -> [w6788]
                      tunnel: w6525 -> [w6787]
                      tunnel: w6524 -> [w6782]
                      tunnel: w6523 -> [w6784]
                      tunnel: w6522 -> [w6786]
                      tunnel: w6521 -> [w6785]
                      tunnel: w6520 -> [w6779]
                      tunnel: w6519 -> [w6780]
                      tunnel: [w6793] -> w6515
                      tunnel: [w6792] -> w6514
                      tunnel: [w6791] -> w6513
                      tunnel: [w6790] -> w6512
                      tunnel: [w6789] -> w6511
                      tunnel: [w6788] -> w6510
                      tunnel: [w6787] -> w6509
                      tunnel: [w6786] -> w6508
                      tunnel: [w6785] -> w6507
                      tunnel: [w6783] -> w6506
                      tunnel: [w6781] -> w6505
                      tunnel: [w6777] -> w6504
                      tunnel: [w6775] -> w6503
                      tunnel: w6518 -> [w6776]
                      tunnel: w6517 -> [w6772]
                      tunnel: [w6771] -> w6502
                      tunnel: w6516 -> [w6771]
                      tunnel: w6515 -> [w6832]
                      tunnel: w6514 -> [w6825]
                      tunnel: w6513 -> [w6816]
                      tunnel: w6512 -> [w6824]
                      tunnel: w6511 -> [w6814]
                      tunnel: w6510 -> [w6823]
                      tunnel: w6509 -> [w6812]
                      tunnel: w6508 -> [w6822]
                      tunnel: w6507 -> [w6810]
                      tunnel: w6506 -> [w6846]
                      tunnel: w6505 -> [w6845]
                      tunnel: w6504 -> [w6821]
                      tunnel: w6503 -> [w6808]
                      tunnel: [w6846] -> w6501
                      tunnel: [w6845] -> w6500
                      tunnel: [w6839] -> w6499
                      tunnel: [w6832] -> w6498
                      tunnel: [w6831] -> w6497
                      tunnel: [w6830] -> w6496
                      tunnel: [w6829] -> w6495
                      tunnel: [w6828] -> w6494
                      tunnel: [w6827] -> w6493
                      tunnel: [w6826] -> w6492
                      tunnel: [w6825] -> w6491
                      tunnel: [w6824] -> w6490
                      tunnel: [w6823] -> w6489
                      tunnel: [w6822] -> w6488
                      tunnel: [w6821] -> w6487
                      tunnel: [w6806] -> w6486
                      tunnel: w6502 -> [w6806]
                      tunnel: [w6859] -> _
                      tunnel: [w6855] -> _
                      tunnel: w6501 -> [w6856]
                      tunnel: w6500 -> [w6859]
                      tunnel: w6499 -> [w6850]
                      tunnel: w6498 -> [w6857]
                      tunnel: w6497 -> [_]
                      tunnel: w6496 -> [_]
                      tunnel: w6495 -> [_]
                      tunnel: w6494 -> [w6847]
                      tunnel: w6493 -> [_]
                      tunnel: w6492 -> [w6851]
                      tunnel: w6491 -> [_]
                      tunnel: w6490 -> [_]
                      tunnel: w6489 -> [_]
                      tunnel: w6488 -> [w6848]
                      tunnel: w6487 -> [_]
                      tunnel: w6486 -> [w6854]
                      frame #0 {
                        w6590 = "%Y-%m-%d" ("time format string (%c)")
                        n1202 = Decimal String To Number(string=w6576) -> (number=w6577:i32)  [unwired: 2 in, 1 out]
                        n1203 = property on="Table" class="Tbl (strict)"("Visible"=TRUE) -> ()  [unwired: 2 in, 2 out]
                        n1204 = Format Date/Time String(time format string (%c)=w6590, seconds (now)=w6582) -> (date/time string=w6591:string)  [unwired: 1 in]
                        n1205 = Format Date/Time String(time format string (%c)=w6590, seconds (now)=w6581) -> (date/time string=w6589:string)  [unwired: 1 in]
                        n1206 = Format Into String(format string="Where BREAKDOWN_DATE between '%s' and '%s' and  SHIFT_ID = '%d'  ", w6591, w6589, w6577) -> (resulting string=w6588:string)  [unwired: 2 in, 1 out]
                        n1207 = call <vilib>:"DB Tools Select Data.vi"("condition"=w6588, "error in (no error)"=w6597, "columns"=string[] ["BREAKDOWN_DATE"], "table"="STATION_1_LOG_HISTORY", "connection reference"=w6599) -> ("error out"=w6584:errorcluster, "data"=w6587:variant[][], "connection reference out"=w6598:T2)  [unwired: 1 in]
                        n1208 = property on="Table 2" class="Tbl (strict)"("Visible"=FALSE) -> ()  [unwired: 2 in, 2 out]
                        n1209 = xnode "Database Variant To Data"("database variant"=w6587, "error in (no error)"=w6584, "type"=string[][] [] ("Elements Found")) -> ("data"=w6585:string[][], "error out"=w6583:errorcluster)
                        n1210 = Index Array(array=w6585, index (col)=0 ("disabled index (col)")) -> (element=w6593:string[])  [unwired: 1 in]
                        n1211 = call "Search_1d_array_element.vi"("Count in"=string[] [] ("Elements Found"), "BD Date"=w6593, "Elements Found in"=string[] [] ("Elements Found")) -> ("Elements Found out"=w6580:string[])  [unwired: 4 in, 2 out]
                        n1212 = Build Array(w6580) -> (w6603:string[][])
                        n1213 = Transpose 2D Array(2D array=w6603) -> (transposed array=w6602:string[][])
                      }
                      frame #1 {
                        n1214 = disable-structure shown="Enabled" {
                          disable-tunnel: w6665 -> [w6676 w6678]
                          disable-tunnel: [w6675 w6678] -> w6664
                          disable-tunnel: w6663 -> [w6674 w6679]
                          disable-tunnel: [w6673 w6679] -> w6662
                          disable-tunnel: w6660 -> [w6671 _]
                          disable-tunnel: w6659 -> [w6670 _]
                          disable-tunnel: [w6669 _] -> w6658
                          disable-tunnel: [w6668 _] -> w6655
                          disable-tunnel: w6653 -> [w6667 _]
                          disable-tunnel: w6650 -> [w6666 w6677]
                          disable-tunnel: [_ w6677] -> w6649
                          frame Disabled {
                            n1215 = call "Stack_holderwise_total_bd_count_&_duration_2.vi"("Refnum in"=w6676, "BREAKDOWN_STK_HOLD_ID"=1, "condition"=w6667, "Form Date"=w6671, "To Date"=w6670, "error in (no error)"=w6674, "Shift"=w6666) -> ("Refnum out"=w6675:T2, "Count out"=w6669:string[], "appended array"=w6668:dbl[], "error out"=w6673:errorcluster)  [unwired: 5 in]
                          }
                          frame Enabled {
                          }
                        }
                        n1216 = call "NUMERIC TO STRING.vi"("appended array"=w6655) -> ("Array"=w6654:string[])  [unwired: 4 in]
                        n1217 = call "Insert_empty_element_with_zero.vi"("searched date"=w6658, "fixed date"=w6656) -> ("O/P"=w6651:string[])  [unwired: 9 in]
                        n1218 = call "Insert_empty_element_with_zero.vi"("searched date"=w6654, "fixed date"=w6656) -> ("O/P"=w6657:string[])  [unwired: 9 in]
                      }
                      frame #2 {
                        n1219 = disable-structure shown="Enabled" {
                          disable-tunnel: w6695 -> [w6709 w6711]
                          disable-tunnel: [w6708 w6711] -> w6694
                          disable-tunnel: w6693 -> [w6707 w6712]
                          disable-tunnel: [w6706 w6712] -> w6692
                          disable-tunnel: w6691 -> [w6705 _]
                          disable-tunnel: w6690 -> [w6704 _]
                          disable-tunnel: [w6703 _] -> w6689
                          disable-tunnel: [w6702 _] -> w6685
                          disable-tunnel: w6683 -> [w6701 _]
                          disable-tunnel: w6681 -> [w6699 w6710]
                          disable-tunnel: [_ w6710] -> w6680
                          frame Disabled {
                            n1220 = call "Stack_holderwise_total_bd_count_&_duration_2.vi"("Refnum in"=w6707, "BREAKDOWN_STK_HOLD_ID"=2, "condition"=w6701, "Form Date"=w6705, "To Date"=w6704, "error in (no error)"=w6709, "Shift"=w6699) -> ("Refnum out"=w6706:T2, "Count out"=w6703:string[], "appended array"=w6702:dbl[], "error out"=w6708:errorcluster)  [unwired: 5 in]
                          }
                          frame Enabled {
                          }
                        }
                        n1221 = call "Insert_empty_element_with_zero.vi"("searched date"=w6689, "fixed date"=w6686) -> ("O/P"=w6688:string[])  [unwired: 9 in]
                        n1222 = call "NUMERIC TO STRING.vi"("appended array"=w6685) -> ("Array"=w6684:string[])  [unwired: 4 in]
                        n1223 = call "Insert_empty_element_with_zero.vi"("searched date"=w6684, "fixed date"=w6686) -> ("O/P"=w6687:string[])  [unwired: 9 in]
                      }
                      frame #3 {
                        n1224 = disable-structure shown="Enabled" {
                          disable-tunnel: w6728 -> [w6744 w6746]
                          disable-tunnel: [w6743 w6746] -> w6727
                          disable-tunnel: w6726 -> [w6742 w6747]
                          disable-tunnel: [w6741 w6747] -> w6725
                          disable-tunnel: w6724 -> [w6740 _]
                          disable-tunnel: w6723 -> [w6739 _]
                          disable-tunnel: [w6738 _] -> w6722
                          disable-tunnel: [w6737 _] -> w6718
                          disable-tunnel: w6716 -> [w6736 _]
                          disable-tunnel: w6714 -> [w6734 w6745]
                          disable-tunnel: [_ w6745] -> w6713
                          frame Disabled {
                            n1225 = call "Stack_holderwise_total_bd_count_&_duration_2.vi"("Refnum in"=w6742, "BREAKDOWN_STK_HOLD_ID"=3, "condition"=w6736, "Form Date"=w6740, "To Date"=w6739, "error in (no error)"=w6744, "Shift"=w6734) -> ("Refnum out"=w6741:T2, "Count out"=w6738:string[], "appended array"=w6737:dbl[], "error out"=w6743:errorcluster)  [unwired: 5 in]
                          }
                          frame Enabled {
                          }
                        }
                        n1226 = call "Insert_empty_element_with_zero.vi"("searched date"=w6722, "fixed date"=w6719) -> ("O/P"=w6721:string[])  [unwired: 9 in]
                        n1227 = call "NUMERIC TO STRING.vi"("appended array"=w6718) -> ("Array"=w6717:string[])  [unwired: 4 in]
                        n1228 = call "Insert_empty_element_with_zero.vi"("searched date"=w6717, "fixed date"=w6719) -> ("O/P"=w6720:string[])  [unwired: 9 in]
                      }
                      frame #4 {
                        n1229 = call "Stack_holderwise_total_bd_count_&_duration_2.vi"("Refnum in"=w6762, "BREAKDOWN_STK_HOLD_ID"=4, "condition"=w6751, "Form Date"=w6759, "To Date"=w6758, "error in (no error)"=w6763, "Shift"=w6748) -> ("Refnum out"=w6761:T2, "Count out"=w6757:string[], "appended array"=w6753:dbl[], "error out"=w6760:errorcluster)  [unwired: 5 in]
                        n1230 = call "Insert_empty_element_with_zero.vi"("searched date"=w6757, "fixed date"=w6754) -> ("O/P"=w6756:string[])  [unwired: 9 in]
                        n1231 = call "NUMERIC TO STRING.vi"("appended array"=w6753) -> ("Array"=w6752:string[])  [unwired: 4 in]
                        n1232 = call "Insert_empty_element_with_zero.vi"("searched date"=w6752, "fixed date"=w6754) -> ("O/P"=w6755:string[])  [unwired: 9 in]
                      }
                      frame #5 {
                        n1233 = disable-structure shown="Enabled" {
                          disable-tunnel: w6784 -> [w6802 w6805]
                          disable-tunnel: [w6801 w6805] -> w6783
                          disable-tunnel: w6782 -> [w6800 w6804]
                          disable-tunnel: [w6799 w6804] -> w6781
                          disable-tunnel: w6780 -> [w6798 _]
                          disable-tunnel: w6779 -> [w6797 _]
                          disable-tunnel: [w6796 _] -> w6778
                          disable-tunnel: [w6795 _] -> w6774
                          disable-tunnel: w6772 -> [w6794 _]
                          frame Disabled {
                            n1234 = call "Stack_holderwise_total_bd_count_&_duration.vi"("Refnum in"=w6800, "BREAKDOWN_STK_HOLD_ID"=5, "condition"=w6794, "Form Date"=w6797, "To Date"=w6798, "error in (no error)"=w6802) -> ("Refnum out"=w6799:T2, "Count out"=w6796:string[], "appended array"=w6795:dbl[], "error out"=w6801:errorcluster)  [unwired: 6 in]
                          }
                          frame Enabled {
                          }
                        }
                        n1235 = call "NUMERIC TO STRING.vi"("appended array"=w6774) -> ("Array"=w6773:string[])  [unwired: 4 in]
                        n1236 = call "Insert_empty_element_with_zero.vi"("searched date"=w6778, "fixed date"=w6776) -> ("O/P"=w6777:string[])  [unwired: 9 in]
                        n1237 = call "Insert_empty_element_with_zero.vi"("searched date"=w6773, "fixed date"=w6776) -> ("O/P"=w6775:string[])  [unwired: 9 in]
                      }
                      frame #6 {
                        n1238 = call "String to numeric.vi"("Array"=w6816) -> ("Array 2"=w6815:dbl[])  [unwired: 4 in]
                        n1239 = call "String to numeric.vi"("Array"=w6814) -> ("Array 2"=w6813:dbl[])  [unwired: 4 in]
                        n1240 = call "String to numeric.vi"("Array"=w6812) -> ("Array 2"=w6811:dbl[])  [unwired: 4 in]
                        n1241 = call "String to numeric.vi"("Array"=w6810) -> ("Array 2"=w6809:dbl[])  [unwired: 4 in]
                        n1242 = call "String to numeric.vi"("Array"=w6808) -> ("Array 2"=w6807:dbl[])  [unwired: 4 in]
                        n1243 = Decimal String To Number(string=w6821) -> (number=w6840:i32[])  [unwired: 2 in, 1 out]
                        n1244 = Decimal String To Number(string=w6822) -> (number=w6841:i32[])  [unwired: 2 in, 1 out]
